vi "freq domain processing.vi"(7 "fft size":u16, 8 "threshold":u16, 9 "input valid":bool, 10 "imag data in":fxp<+/-,28,16>, 11 "real data in":fxp<+/-,28,16>) -> (1 "output valid":bool, 2 "imag data out":fxp<+/-,28,16>, 3 "real data out":fxp<+/-,28,16>)   [LabVIEW 2020]
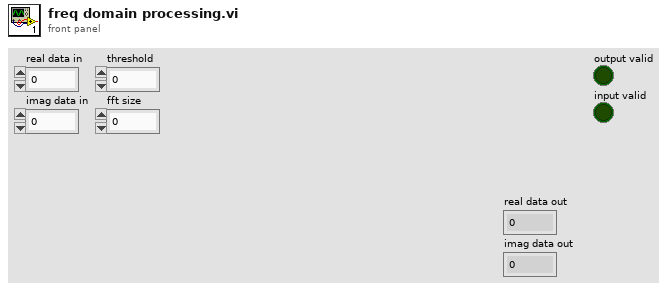
[diagram p1: front panel]
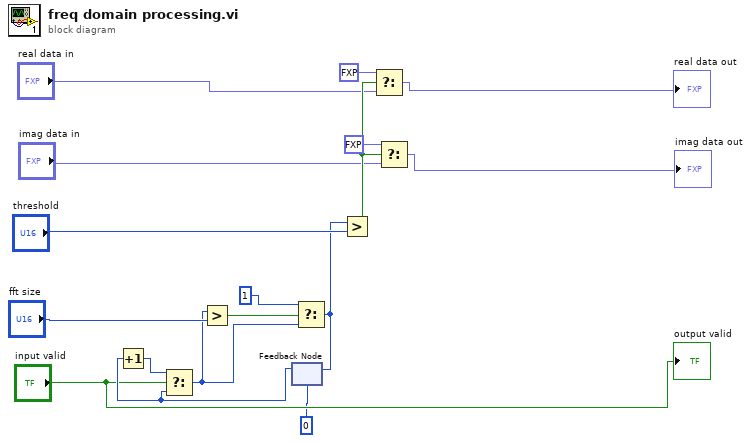
[diagram p0: block diagram]
diagram:
  n1 = feedback #1(u16 0) -> (w13:u16)
  n2 = Increment(x=w13) -> (x+1=w14:u16)
  n3 = Select(t=w14, s="input valid", f=w13) -> (s? t:f=w12:u16)
  n4 = Greater?(x=w12, y="fft size") -> (0:w16:bool)
  n5 = Select(t=u16 1, s=w16, f=w12) -> (s? t:f=w10:u16)
  n6 = feedback-in #1(w10) -> ()
  n7 = Greater?(x=w10, y="threshold") -> (0:w9:bool)
  n8 = Select(t=fxp<+/-,28,16> 0.0, s=w9, f="real data in") -> (s? t:f=→"real data out":fxp<+/-,28,16>)
  n9 = Select(t=fxp<+/-,28,16> 0.0, s=w9, f="imag data in") -> (s? t:f=→"imag data out":fxp<+/-,28,16>)
  "output valid" <- "input valid"
